vi "CalculateDeviceFeatures.vi"(8 "error in (no error)":errorcluster, 9 "Map":T2, 10 "Waveforms":T1, 11 "Group":T3) -> (0 "error out":errorcluster, 3 "Group out":T3)   [LabVIEW 2017, in "CmsAnalysis.lvlib"]
uses:
  <vilib>/addons/InsightCM/Devices/Shared/Cms/CmsAnalysis/CmsAnalysis.lvlib
  <vilib>/addons/PointValueMap/controls/PointMap.ctl
  <vilib>/addons/InsightCM/Devices/Shared/Cms/CmsAnalysis/controls/Group.ctl
  <vilib>/addons/InsightCM/Utilities/Analysis/Shared/controls/Channel.ctl
  <vilib>/addons/InsightCM/Utilities/Analysis/Shared/controls/SpeedType.ctl
  <vilib>/addons/InsightCM/Utilities/Analysis/Shared/controls/Feature.ctl
  <vilib>/addons/InsightCM/Utilities/Analysis/Shared/controls/AmplitudeScale.ctl
  <vilib>/addons/InsightCM/Utilities/DataAccessors/controls/wfmSGL_DVR.ctl
  <vilib>/addons/InsightCM/Utilities/Analysis/Shared/AnalysisHelper.lvlib
  <vilib>/addons/PointValueMap/PointValueMap.lvlib
panel:
  out "data flow map out":T2
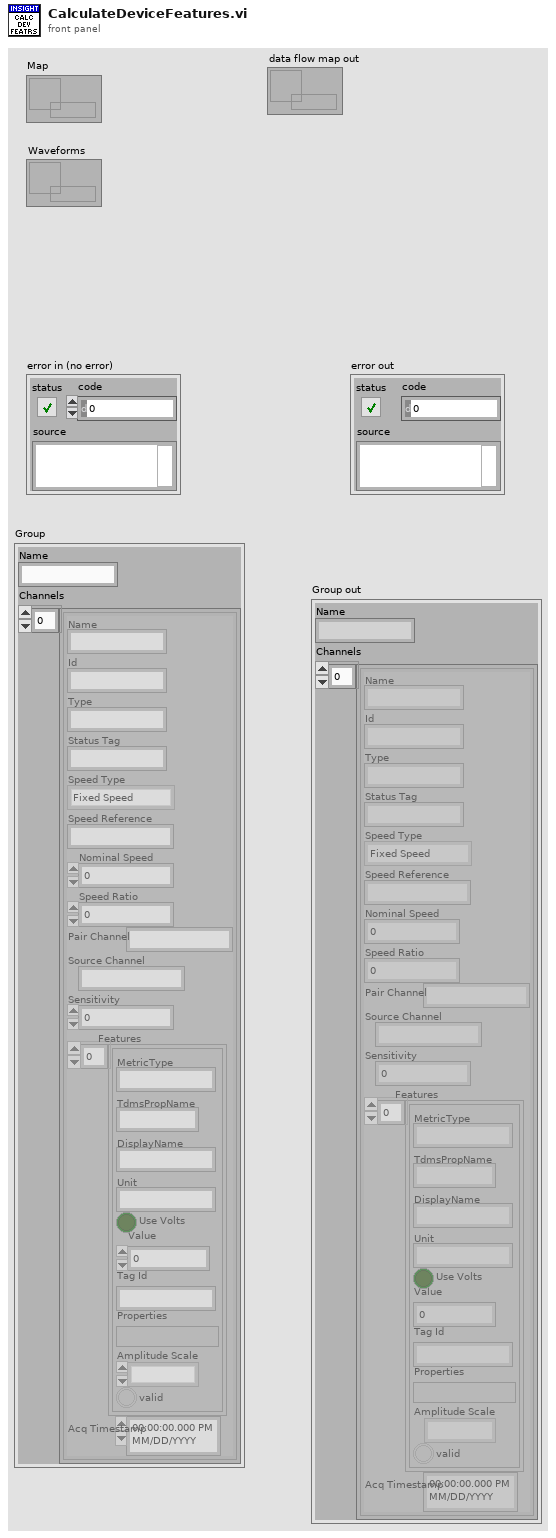
[diagram p1: front panel]
types:
  T1 = typedef "wfmSGL_DVR.ctl" = refnum<data-value>
  T2 = typedef "PointValueMap.lvlib/PointMap.ctl" = refnum<data-value>
  T3 = typedef "CmsAnalysis.lvlib/Group.ctl" = cluster{"Name":string, "Channels":T4[]}
  T4 = typedef "AnalysisHelper.lvlib/Channel.ctl" = cluster{"Name":string, "Id":string, "Type":string, "Status Tag":string, "Speed Type":T5, "Speed Reference":string, "Nominal Speed":dbl, "Speed Ratio":dbl, "Pair Channel":string, "Source Channel":string, "Sensitivity":dbl, "Features":T6[], "Acq Timestamp":timestamp}
  T5 = typedef "AnalysisHelper.lvlib/SpeedType.ctl" = enum16{"Fixed Speed", "Tachometer", "From Map"}
  T6 = typedef "AnalysisHelper.lvlib/Feature.ctl" = cluster{"MetricType":string, "TdmsPropName":string, "DisplayName":string, "Unit":string, "Use Volts":bool, "Value":dbl, "Tag Id":string, "Properties":variant, "Amplitude Scale":T7, "valid":bool}
  T7 = typedef "AnalysisHelper.lvlib/AmplitudeScale.ctl" = enum16{"rms", "peak", "pk-pk"}
  T8 = typedef "AnalysisHelper.lvlib/PulsePositions.ctl" = cluster{"Name":string, "Pulse Position Data":dbl[], "Pulses Per Rev":i32}
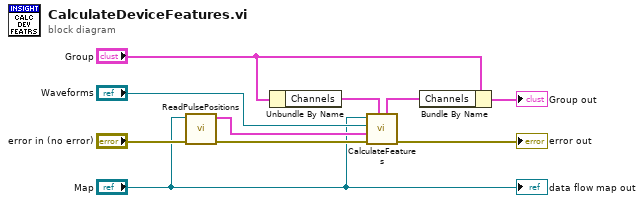
[diagram p0: block diagram]
diagram:
  n1 = call <vilib>:"ReadPulsePositions.vi"("error in (no error)"="error in (no error)", "Map"="Map") -> ("error out"=w6:errorcluster, "pulse positions array"=w8:T8[])  [unwired: 7 in, 1 out]
  n2 = Unbundle By Name("Group") -> ("Channels"=w3:T4[])
  n3 = call <vilib>:"CalculateFeatures.vi"("channels"=w3, "error in (no error)"=w6, "pulse positions array"=w8, "waveforms"="Waveforms", "Map"="Map") -> ("error out"=→"error out":errorcluster, "channels out"=w2:T4[])  [unwired: 5 in]
  n4 = Bundle By Name(cluster="Group", "Channels"=w2) -> (→"Group out":T3)
  "data flow map out" <- "Map"
